vi "PicoScope2000NearestSampleInterval.vi"(5 "Enabled Array":i16[](array[numeric]), 6 "Acquisition Settings":T1 {"postTriggerSamples" format="%_6p"; "preTriggerSamples" format="%_6p"}, 8 "error in (no error)":errorcluster, 9 "roundFaster":bool, 10 "timeIntervalRequested":dbl format="%#6_6p", 11 "handle in":i16) -> (0 "error out":errorcluster, 1 "timebase":i16, 2 "timeIntervalAvailable":dbl format="%#6_6p", 3 "handle out":i16)   [LabVIEW 2010]
doc: "Calls Gettimebase function"
uses:
  ps2000.dll
  shared/Acquisition Settings.ctl
panel:
  in  "Memory Segment":u32
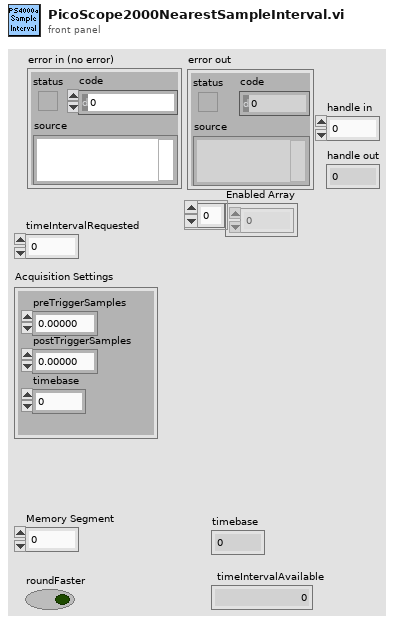
[diagram p1: front panel]
types:
  T1 = typedef "Acquisition Settings.ctl" = cluster{"preTriggerSamples":u64, "postTriggerSamples":u64, "timebase":u32}
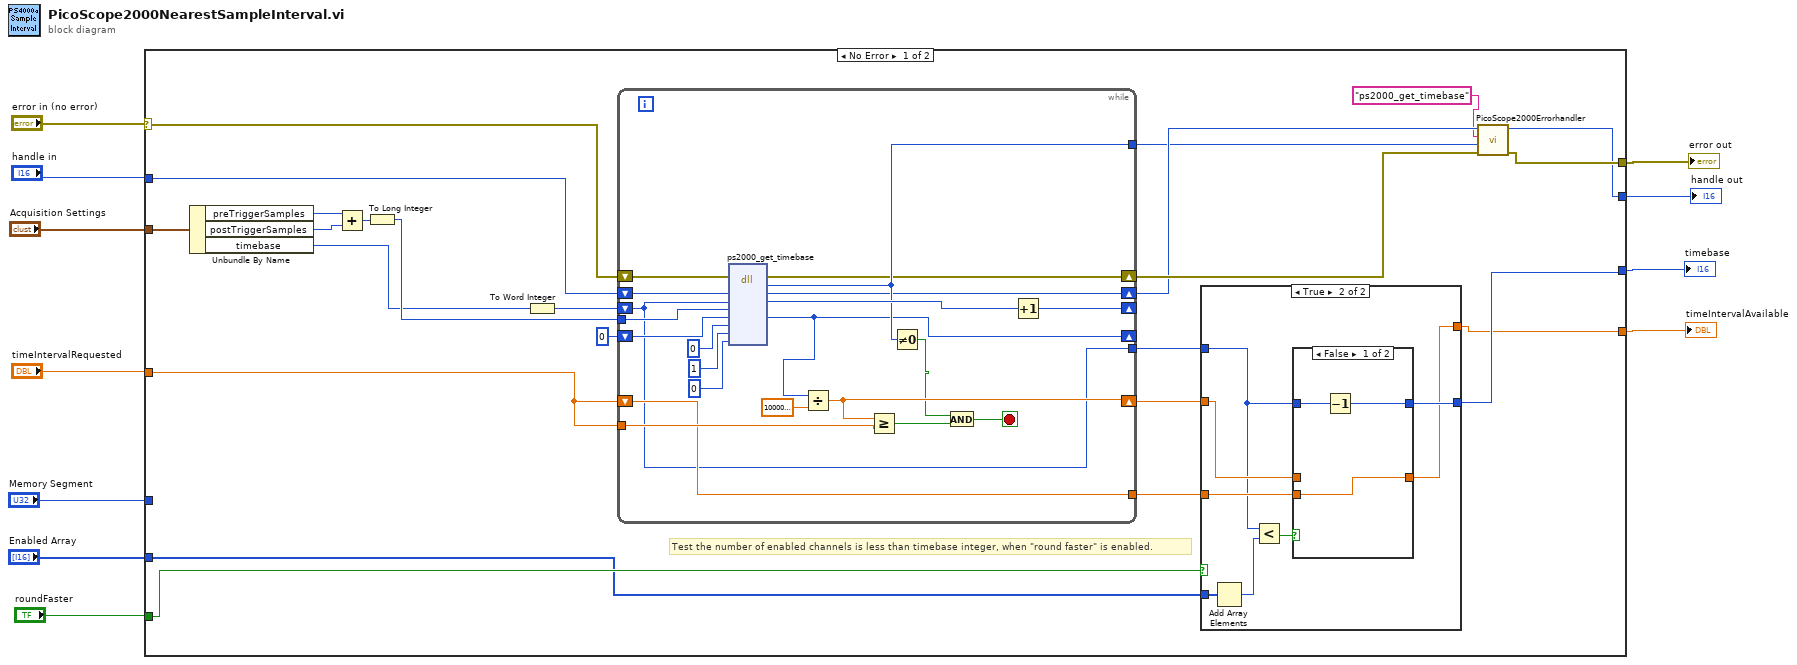
[diagram p0: block diagram]
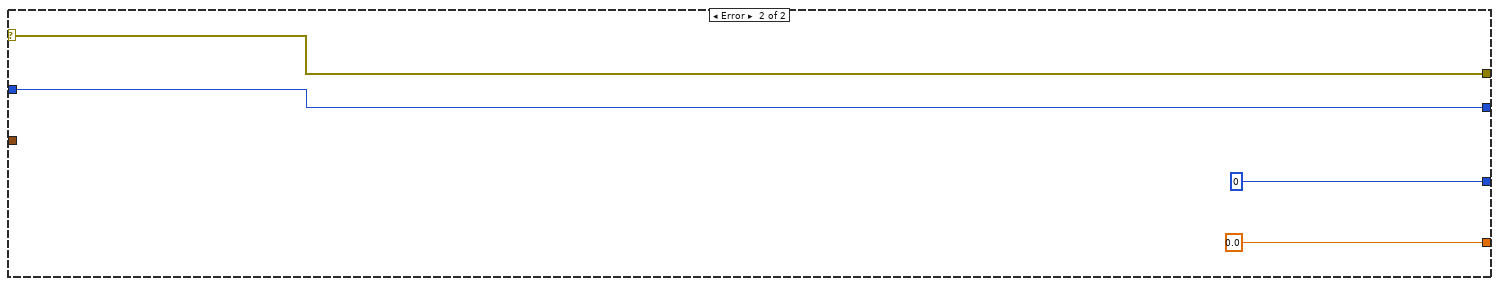
[diagram p4: hidden frame]
diagram:
  n1 = case shown="No Error" "error in (no error)" {
    selector: "error in (no error)" -> [w30 w75]
    tunnel: [w25 w75] -> w11
    tunnel: [w24 w74] -> w10
    tunnel: "handle in" -> [w31 w74]
    tunnel: "roundFaster" -> [w16 _]
    tunnel: "timeIntervalRequested" -> [w17 _]
    tunnel: [w26 i16 0 ("timebase")] -> w5
    tunnel: [w20 0.0 ("timeIntervalAvailable")] -> w4
    tunnel: "Acquisition Settings" -> [w32 _]
    tunnel: "Memory Segment" -> [_ _]
    tunnel: "Enabled Array" -> [w15 _]
    frame No Error {
      # "Test the number of enabled channels is less than timebase integer, when \"round faster\" is enabled."
      n2 = Unbundle By Name(w32) -> ("preTriggerSamples"=w34:u64, "postTriggerSamples"=w35:u64, "timebase"=w12:u32)
      n3 = Add(x=w34, y=w35) -> (x+y=w33:u64)
      n4 = To Long Integer(number=w33) -> (32bit integer=w19:i32)
      n5 = To Word Integer(number=w12) -> (16bit integer=w13:i16)
      n6 = while {
        tunnel: w19 -> [w62]
        shift-right: [w58] -> w22
        shift-left: w31 -> [w68]
        shift-right: [w59] -> w23
        shift-left: w30 -> [w69]
        shift-right: [w52] -> _
        shift-left: w13 -> [w51]
        tunnel: w17 -> [w71]
        shift-right: [w65] -> w28
        shift-left: w17 -> [w70]
        tunnel: [w70] -> w29
        tunnel: [w51] -> w27
        tunnel: [w60] -> w21
        shift-right: [w56] -> _
        shift-left: 0 ("time_interval") -> [w57]
        stop <- w55 stop-if-true
        n7 = dll-call lib="PS2000.dll" fn="ps2000_get_timebase"(error in=w69, "handle"=w68, "timebase"=w51, "no_of_samples"=w62, "time_interval"=w57, "time_units"=i16 0, "oversample"=i16 1, "max_sample"=0 ("maxSamples")) -> (error out=w59:errorcluster, "return type"=w60:i16, "handle"=w58:i16, "timebase"=w67:i16, "time_interval"=w56:i32)  [unwired: 6 in, 1 out]
        n8 = Divide(x=w56, y=1000000000.0) -> (x/y=w65:dbl)
        n9 = Greater Or Equal?(x=w65, y=w71) -> (x >= y?=w54:bool)
        n10 = Not Equal To 0?(x=w60) -> (x != 0?=w53:bool)
        n11 = And(x=w53, y=w54) -> (x .and. y?=w55:bool)
        n12 = Increment(x=w67) -> (x+1=w52:i16)
      }
      n13 = case shown="True" w16 {
        tunnel: [w37 w44] -> w20
        tunnel: w29 -> [_ w43]
        tunnel: w28 -> [w37 w42]
        tunnel: [w36 w45] -> w26
        tunnel: w27 -> [w36 w40]
        tunnel: w15 -> [_ w39]
        frame False {
        }
        frame True {
          n14 = Add Array Elements(numeric array=w39) -> (sum=w38:i16)
          n15 = Less?(x=w40, y=w38) -> (x < y?=w41:bool)
          n16 = case shown="False" w41 {
            tunnel: [w48 w50] -> w45
            tunnel: w40 -> [w47 w50]
            tunnel: [w46 w49] -> w44
            tunnel: w43 -> [w46 _]
            tunnel: w42 -> [_ w49]
            frame False {
              n17 = Decrement(x=w47) -> (x-1=w48:i16)
            }
            frame True {
            }
          }
        }
      }
      n18 = call "PicoScope2000Errorhandler.vi"("Handle in"=w22, "API function"="ps2000_get_timebase" ("source"), "Return"=w21, "error in (no error)"=w23) -> ("Handle out"=w24:i16, "error out"=w25:errorcluster)  [unwired: 5 in]
    }
    frame Error {
    }
  }
  "error out" <- w11
  "handle out" <- w10
  "timebase" <- w5
  "timeIntervalAvailable" <- w4
